vi "test json to variant uint.vi"(8 "error in (no error)":errorcluster) -> (0 "error out":errorcluster)   [LabVIEW 2019, in "labview_json_tests.lvlib"]
uses:
  labview_json_tests.lvlib
  lib/labview_json.lvlib
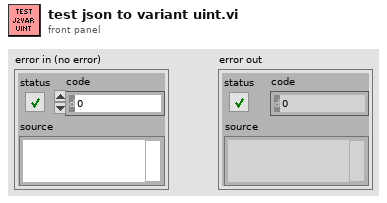
[diagram p1: front panel]
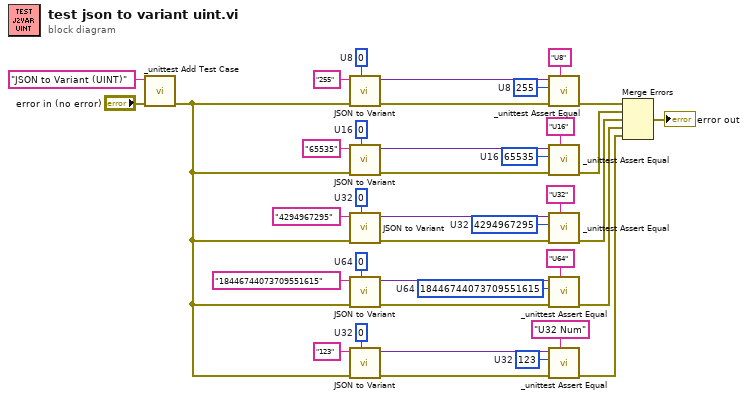
[diagram p0: block diagram]
diagram:
  w8 = u32 123  # U32
  w7 = u32 0  # U32
  w11 = u64 18446744073709551615  # U64
  w12 = u64 0  # U64
  w22 = u32 4294967295  # U32
  w21 = u32 0  # U32
  w23 = u16 65535  # U16
  w24 = u16 0  # U16
  w25 = u8 255  # U8
  w26 = u8 0  # U8
  n1 = call "_unittest Add Test Case.vi"("error in (no error)"="error in (no error)", "Test Case"="JSON to Variant (UINT)") -> ("error out"=w1:errorcluster)  [unwired: 9 in]
  n2 = call "JSON to Variant.vi"("Variant Type"=w26, "error in (no error)"=w1, "JSON"="255") -> ("error out"=w34:errorcluster, "Variant out"=w32:variant)  [unwired: 7 in]
  n3 = call "JSON to Variant.vi"("Variant Type"=w24, "error in (no error)"=w1, "JSON"="65535") -> ("error out"=w29:errorcluster, "Variant out"=w31:variant)  [unwired: 7 in]
  n4 = call "JSON to Variant.vi"("Variant Type"=w21, "error in (no error)"=w1, "JSON"="4294967295") -> ("error out"=w19:errorcluster, "Variant out"=w17:variant)  [unwired: 7 in]
  n5 = call "JSON to Variant.vi"("Variant Type"=w12, "error in (no error)"=w1, "JSON"="18446744073709551615") -> ("error out"=w14:errorcluster, "Variant out"=w16:variant)  [unwired: 7 in]
  n6 = call "JSON to Variant.vi"("Variant Type"=w7, "error in (no error)"=w1, "JSON"="123") -> ("error out"=w5:errorcluster, "Variant out"=w3:variant)  [unwired: 7 in]
  n7 = call "_unittest Assert Equal.vi"("Message"="U8", "error in (no error)"=w34, "Expected Value"=w25, "Actual Value"=w32) -> ("error out"=w37:errorcluster)  [unwired: 7 in]
  n8 = call "_unittest Assert Equal.vi"("Message"="U16", "error in (no error)"=w29, "Expected Value"=w23, "Actual Value"=w31) -> ("error out"=w27:errorcluster)  [unwired: 7 in]
  n9 = call "_unittest Assert Equal.vi"("Message"="U32", "error in (no error)"=w19, "Expected Value"=w22, "Actual Value"=w17) -> ("error out"=w10:errorcluster)  [unwired: 7 in]
  n10 = call "_unittest Assert Equal.vi"("Message"="U64", "error in (no error)"=w14, "Expected Value"=w11, "Actual Value"=w16) -> ("error out"=w9:errorcluster)  [unwired: 7 in]
  n11 = call "_unittest Assert Equal.vi"("Message"="U32 Num", "error in (no error)"=w5, "Expected Value"=w8, "Actual Value"=w3) -> ("error out"=w2:errorcluster)  [unwired: 7 in]
  n12 = Merge Errors(w37, w27, w10, w9, w2) -> (→"error out":errorcluster)
